vi "PH_Powermeter_BaseClass.PC Set Scaling Factor.vi"(0 "VI in":refnum<vi>, 2 "Scaling Factor":dbl=1.0, 5 "error in (no error)":errorcluster) -> (14 "VI out":refnum<vi>, 19 "error out":errorcluster)   [LabVIEW 2014, in "PH_Powermeter_BaseClass.lvlib"]
doc: "If the incoming value is not zero and deiffers from stored value, the scaling factor is set to own attributtes. Aferwards, the energy is recalculated and set as well to own attributes as to GUI and DIM service."
uses:
  PH_Powermeter_BaseClass.lvlib
  PH_Common/PH_Common.lvlib
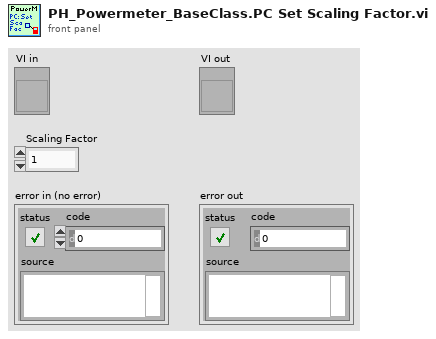
[diagram p1: front panel]
types:
  T1 = typedef "PH_Powermeter_BaseClass.lvlib/PH_Powermeter_BaseClass.i attribute.ctl" = cluster{"GUI References":T2, "Connection":T3, "Head Attributes":T5, "VISA resource":refnum<visa-resource-name>, "Energy":T6, "Service ID Energy":i32, "Wanted Settings":T7, "Current Settings":T7}
  T2 = typedef "PH_Powermeter_BaseClass.lvlib/PH_Powermeter_BaseClass.GUI Refs.ctl" = cluster{"Head Attributes":refnum<vi>, "Energy":refnum<vi>, "Connection":refnum<vi>, "VISA Resource":refnum<vi>, "Scaling Factor":refnum<vi>, "Range":refnum<vi>, "Wavelength":refnum<vi>, "Trigger Level":refnum<vi>, "Wanted Settings":refnum<vi>, "Current Settings":refnum<vi>}
  T3 = typedef "PH_Powermeter_BaseClass.lvlib/PH_Powermeter_BaseClass.Connection.ctl" = cluster{"failed checks":i8, "Timeout":bool, "Data read":string, "Failure":bool, "Error":bool, "State":T4}
  T4 = typedef "PH_Powermeter_BaseClass.lvlib/PH_Powermeter_BaseClass.State.ctl" = enum32{"off", "operating", "opened", "checked", "connected", "Sets to change", "running"}
  T5 = typedef "PH_Powermeter_BaseClass.lvlib/PH_Powermeter_BaseClass.Head Attributes.ctl" = cluster{"Instrument Type":string, "Head Version":string, "Head Name":string, "Serial Number":string, "Firmware":string, "Sensor Type":string, "MinimumRange":u32, "Maximum Range":u32, "Min Wavelength":i32, "Max Wavelength":i32}
  T6 = typedef "PH_Powermeter_BaseClass.lvlib/PH_Powermeter_BaseClass.Energy.ctl" = cluster{"current Value":dbl, "unscaled":dbl, "Scaling Factor":dbl}
  T7 = typedef "PH_Powermeter_BaseClass.lvlib/PH_gentec_BaseClass.Head Settings.ctl" = cluster{"Trigger Level":dbl, "Wavelength":u32, "Range":u32}
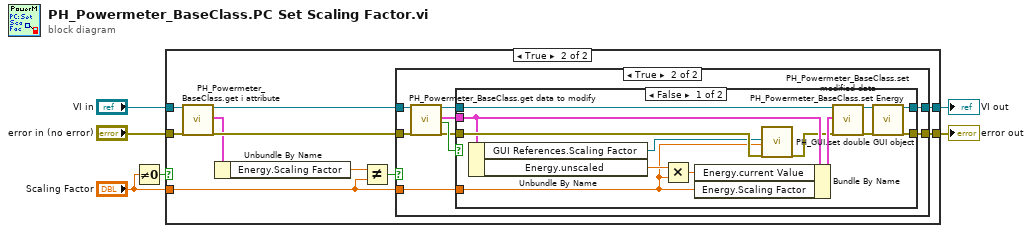
[diagram p0: block diagram]
diagram:
  n1 = Not Equal To 0?(x="Scaling Factor") -> (x != 0?=w1:bool)
  n2 = case shown="True" w1 {
    tunnel: [w7 w18] -> w6
    tunnel: "error in (no error)" -> [w7 w17]
    tunnel: [w8 w16] -> w4
    tunnel: "VI in" -> [w8 w14]
    tunnel: "Scaling Factor" -> [_ w10]
    frame False {
    }
    frame True {
      n3 = call "PH_Powermeter_BaseClass.get i attribute.vi"("i ref in"=w14, "error in (no error)"=w17) -> ("i ref out"=w13:refnum<vi>, "i attribute"=w12:T1, "error out"=w15:errorcluster)  [unwired: 15 in]
      n4 = Unbundle By Name(w12) -> ("Energy.Scaling Factor"=w11:dbl)
      n5 = Not Equal?(x=w11, y=w10) -> (x != y?=w9:bool)
      n6 = case shown="True" w9 {
        tunnel: [w19 w27] -> w18
        tunnel: [w20 w25] -> w16
        tunnel: w15 -> [w19 w23]
        tunnel: w13 -> [w20 w22]
        tunnel: w10 -> [_ w21]
        frame False {
        }
        frame True {
          n7 = call "PH_Powermeter_BaseClass.get data to modify.vi"("i ref in"=w22, "error in (no error)"=w23) -> ("i ref out"=w24:refnum<vi>, "i attribute"=w29:T1, "timed out"=w28:bool, "error out"=w26:errorcluster)  [unwired: 14 in]
          n8 = case shown="False" w28 {
            tunnel: w24 -> [w42 w44]
            tunnel: [w38 w44] -> w25
            tunnel: w26 -> [w41 w43]
            tunnel: [w36 w43] -> w27
            tunnel: w29 -> [w35 _]
            tunnel: w21 -> [w30 _]
            frame False {
              n9 = Unbundle By Name(w35) -> ("GUI References.Scaling Factor"=w31:refnum<vi>, "Energy.unscaled"=w34:dbl)
              n10 = Multiply(x=w34, y=w30) -> (x*y=w33:dbl)
              n11 = Bundle By Name(cluster=w35, "Energy.current Value"=w33, "Energy.Scaling Factor"=w30) -> (w40:T1)
              n12 = call "PH_GUI.set double GUI object.vi"("GUI object Ref"=w31, "value"=w30, "error in (no error)"=w41) -> ("error out"=w32:errorcluster)  [unwired: 16 in]
              n13 = call "PH_Powermeter_BaseClass.set modified data.vi"("i ref in"=w42, "i attribute"=w40, "error in (no error)"=w32) -> ("i ref out"=w39:refnum<vi>, "error out"=w37:errorcluster)  [unwired: 15 in]
              n14 = call "PH_Powermeter_BaseClass.set Energy.vi"("VI in"=w39, "error in (no error)"=w37) -> ("VI out"=w38:refnum<vi>, "error out"=w36:errorcluster)  [unwired: 16 in]
            }
            frame True {
            }
          }
        }
      }
    }
  }
  "error out" <- w6
  "VI out" <- w4
